vi "sicm_main.vi"(6 "sicm.blc.p.params":T8={"se.blc.p.postRetractDelay"=0, "se.blc.p.windowSize"=0, "se.blc.p.updateFactor"=-8, "blc.resetBackground"=FALSE, "se.blc.p.mindelta"=0.0}, 7 "sicm.display":T4, 8 "sicm.p.clocks":T10, 9 "sicm.p.params":T2={"sicm.p.setPoint"=0.9999847412109375, "sicm.p.setPointFrac"=1.0, "stepDown"=0.0, "retractHeight"=0.0, "adaptiveMin"=0.0} {"sicm.p.setPoint" format="%#_3g"}, 10 "sicm.p.modes":T9, 11 "sicm.i.current":T6) -> (0 "sicm.debug":T3, 1 "sicm.s.baseline":T1, 2 "sicm.triggerHeight":T7, 3 "heightOut":T5)   [LabVIEW 2016]
uses:
  <vilib>/rvi/FXPMathLib/FxpDiv/subVIs/nifxpmath_Div_SimConfig.ctl
  <vilib>/rvi/Emulation/niFpgaEmulationIsFPGAContextNoSignature.vi
  <vilib>/rvi/Emulation/niFpgaSctlEmulationGetInTimedLoop.vi
  <vilib>/rvi/errors/niFpgaSetErrorForExecOnDevCompSimple.vi
  <vilib>/rvi/eio/common/nirviEmuReportErrorAndStop.vi
  <vilib>/rvi/DataTransferAndStorage/Container/Common/niFpgaContainerGetUniqueNameForEmu.vi
  <vilib>/rvi/FIFO/Fifo_Resource/nirvififoEmulationSetSize.vi
  <vilib>/rvi/FIFO/Fifo_Resource/nirviFifoEmulationQueueMgr.vi
  <instcachedir>/0/nirviFifoEmulationQueueMgr_E5CAEC123FF24DC58D834DCA3CDAA9B5.lvgen/nirviFifoEmulationQueueMgr_E5CAEC123FF24DC58D834DCA3CDAA9B5_033.vi
  <vilib>/rvi/FIFO/Fifo_Resource/nirvififoEmulationDetermineInputValidOut.vi
  <vilib>/rvi/FIFO/Fifo_Resource/nirvififoEmulationCreateLock.vi
  <vilib>/rvi/Emulation/niFpgaProcessEmulError.vi
  <vilib>/rvi/FIFO/Fifo_Resource/nirvififoEmulationObtainLock.vi
  <vilib>/rvi/FIFO/Fifo_Resource/nirvififoEmulationReleaseLock.vi
  <vilib>/rvi/occurrence/nirviWaitOnOccurrenceBase.vi
  <vilib>/rvi/errors/nirviReportUnexpectedCaseInternalError.vi
  <vilib>/rvi/errors/nirviReportUnexpectedCaseInternalError (U32).vi
  <vilib>/rvi/FXPMathLib/FxpDiv/simVIs/DllFxpDivTemp_sub.vi
  <instrlib>/_niInstr/Basic Elements/v1/FPGA/Private/Count Down U8.vi
  <vilib>/rvi/FXPMathLib/FxpInterpret/XNode/nifxpmath_Interpret.xnode
  <vilib>/rvi/DataTransferAndStorage/Container/XNode/niFpgaContainer.xnode
  <vilib>/rvi/FIFO/Fifo_Resource/nirvififoEmulationWrite.vi
  <vilib>/rvi/FXPMathLib/FxpMul/XNode/nifxpmath_Multiplier.xnode
  <vilib>/rvi/FXPMathLib/FxpSub/XNode/nifxpmath_Sub.xnode
  <vilib>/rvi/FXPMathLib/FxpReciprocal/XNode/nifxpmath_Reciprocal.xnode
  <vilib>/rvi/FXPMathLib/FxpDiv/XNode/nifxpmath_Div.xnode
  <vilib>/rvi/DataTransferAndStorage/Handshake/Emulation/niFpgaHandshakeEmulation.vi
  <vilib>/rvi/FXPMathLib/FxpAdd/XNode/nifxpmath_Add.xnode
  <vilib>/rvi/FXPMathLib/sim/FxpSim.dll
  <instrlib>/_niInstr/Basic Elements/v1/FPGA/niInstr Basic Elements v1 FPGA.lvlib
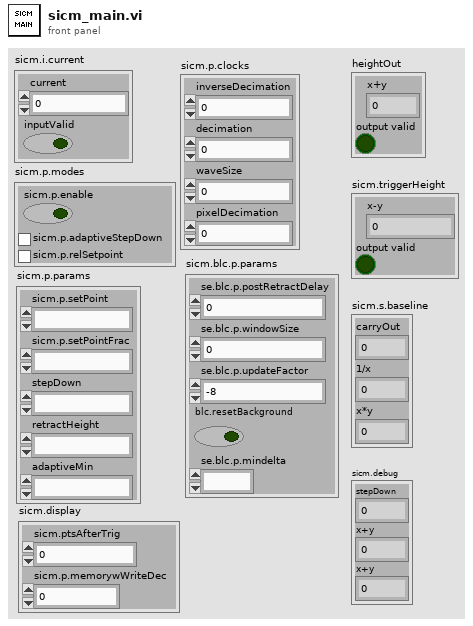
[diagram p1: front panel]
types:
  T1 = cluster{"carryOut":fxp<+/-,22,2>, "1/x":fxp<+/-,32,24>, "x*y":fxp<+,24,1>}
  T2 = cluster{"sicm.p.setPoint":fxp<+,20,0>, "sicm.p.setPointFrac":fxp<+/-,20,14>, "stepDown":fxp<+/-,28,4>, "retractHeight":fxp<+/-,28,4>, "adaptiveMin":fxp<+,10,0>}
  T3 = cluster{"stepDown":fxp<+/-,28,4>, "x+y":fxp<+/-,20,1>, "x+y":fxp<+/-,28,1>}
  T4 = cluster{"sicm.ptsAfterTrig":u16, "sicm.p.memorywWriteDec":u16}
  T5 = cluster{"x+y":fxp<+/-,28,2>, "output valid":bool}
  T6 = cluster{"current":fxp<+/-,24,16>, "inputValid":bool}
  T7 = cluster{"x-y":fxp<+/-,22,4>, "output valid":bool}
  T8 = cluster{"se.blc.p.postRetractDelay":u16, "se.blc.p.windowSize":u16, "se.blc.p.updateFactor":i16, "blc.resetBackground":bool, "se.blc.p.mindelta":fxp<+/-,12,-14>}
  T9 = cluster{"sicm.p.enable":bool, "sicm.p.adaptiveStepDown":bool, "sicm.p.relSetpoint":bool}
  T10 = cluster{"inverseDecimation":fxp<+,22,0>, "decimation":u16, "waveSize":u16, "pixelDecimation":u16}
  T11 = cluster{"address":u16, "interactionPair":cluster{"Current":i16, "Height":i16}}
  T12 = cluster{"upper limit":fxp<+/-,29,2>, "edge detected":bool}
  T13 = cluster{"current":fxp<+/-,24,16>, "y":fxp<+/-,29,16>}
  T14 = cluster{"carryOut":fxp<+/-,28,2>, "1/x":fxp<+/-,32,24>, "x*y":fxp<+,24,1>}
  T15 = cluster{"stepDown":fxp<+/-,28,4>, "upper limit":fxp<+/-,29,2>, "x+y":fxp<+/-,29,2>}
  T16 = cluster{"x+y":fxp<+/-,29,2>, "output valid":bool}
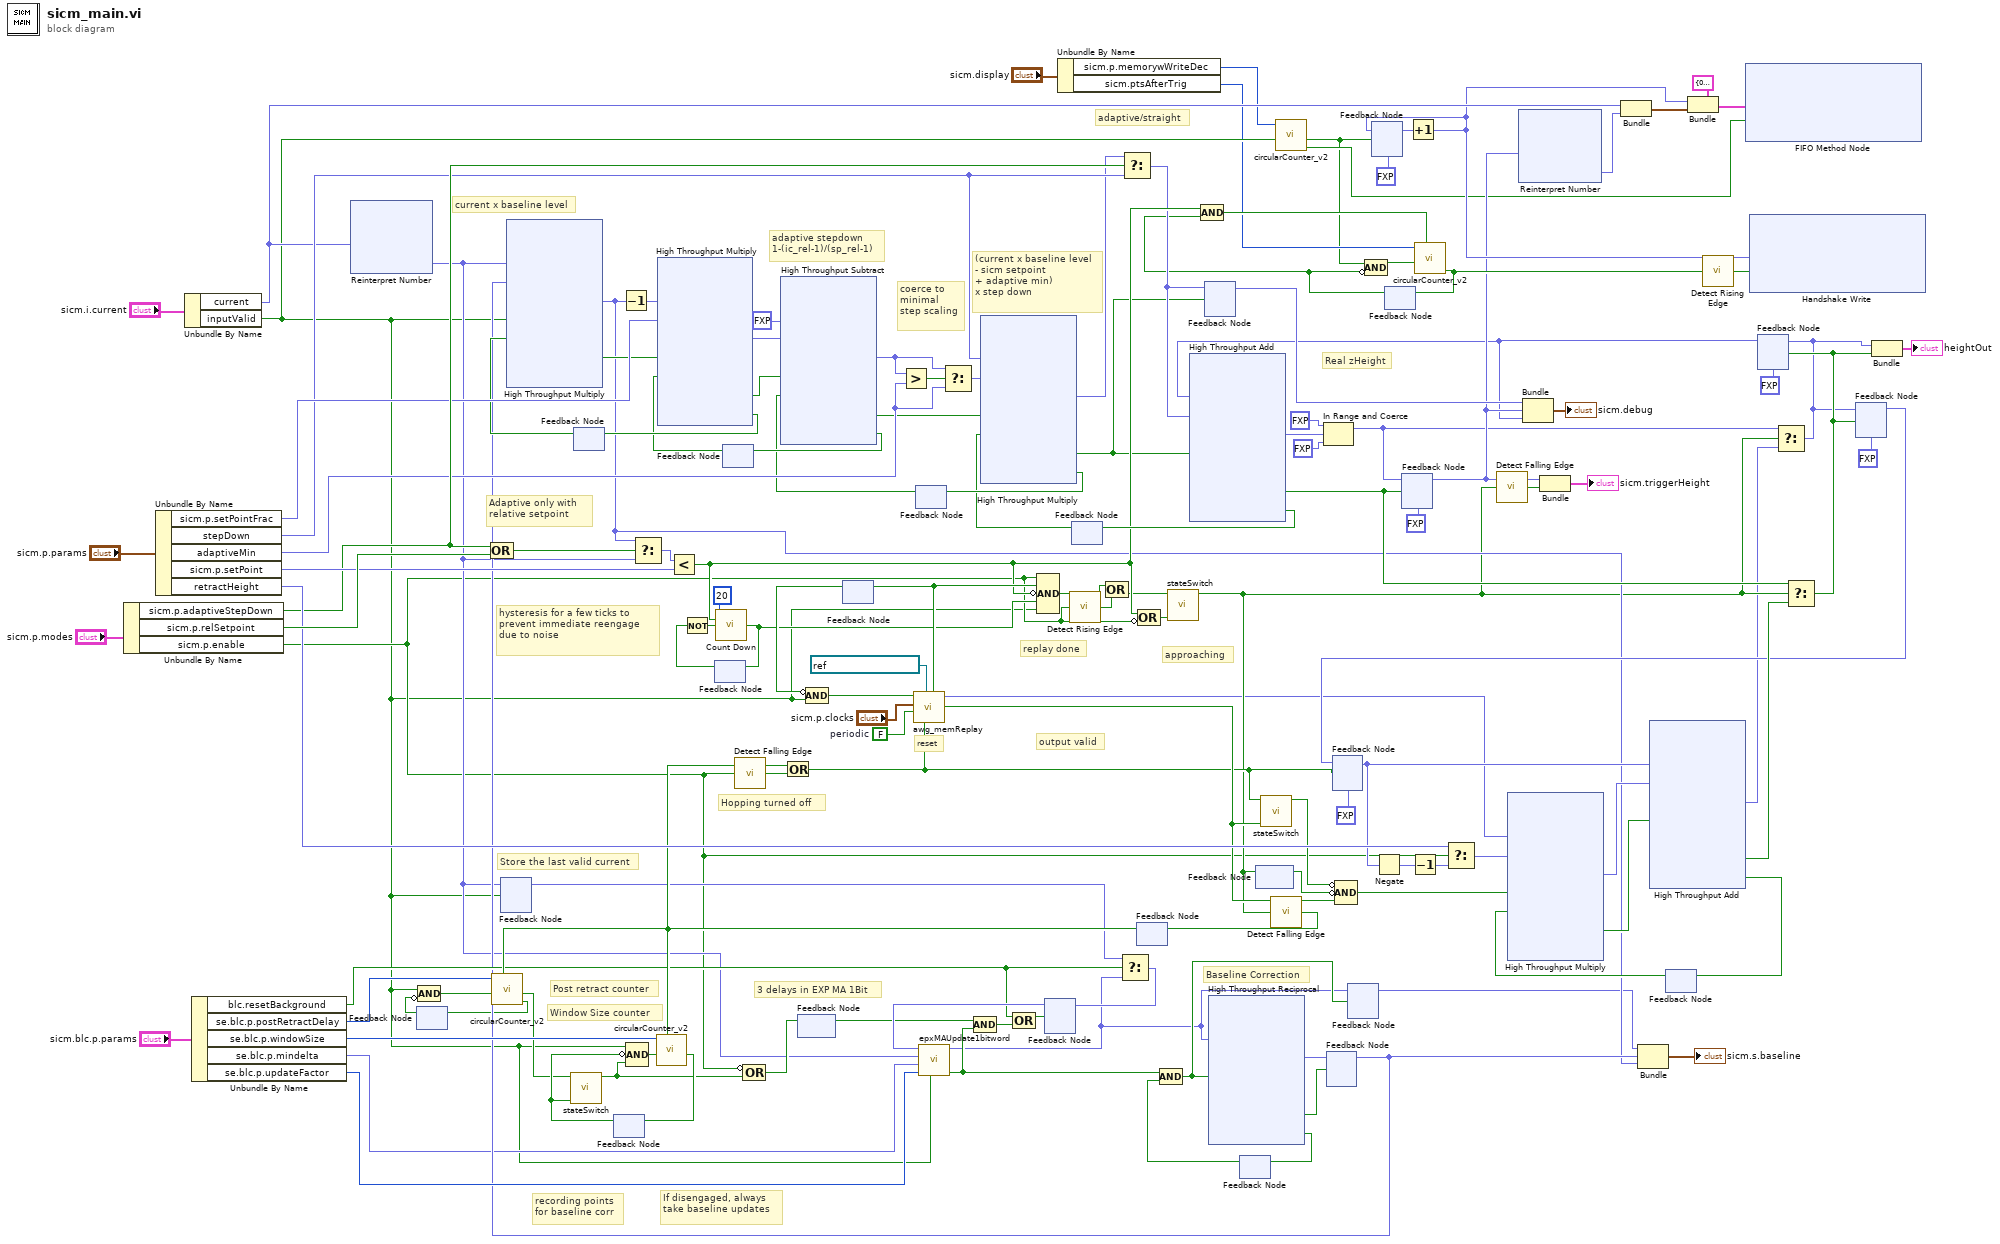
[diagram p0: block diagram]
diagram:
  w135 = FALSE  # periodic
  # "3 delays in EXP MA 1Bit"
  # "Window Size counter"
  # "Post retract counter"
  # "Hopping turned off"
  # "Store the last valid current"
  # "hysteresis for a few ticks to prevent immediate reengage due to noise"
  # "adaptive stepdown\n1-(ic_rel-1)/(sp_rel-1)"
  # "coerce to minimal step scaling"
  # "replay done"
  # "output valid"
  # "reset"
  # "(current x baseline level \n- sicm setpoint \n+ adaptive min)\nx step down"
  # "current x baseline level"
  # "If disengaged, always take baseline updates"
  # "Adaptive only with \nrelative setpoint"
  # "recording points\nfor baseline corr"
  # "Baseline Correction"
  # "adaptive/straight"
  # "approaching"
  # "Real zHeight"
  n1 = Unbundle By Name("sicm.p.modes") -> ("sicm.p.adaptiveStepDown"=w111:bool, "sicm.p.relSetpoint"=w120:bool, "sicm.p.enable"=w22:bool)
  n2 = Unbundle By Name("sicm.p.params") -> ("sicm.p.setPointFrac"=w104:fxp<+/-,20,14>, "stepDown"=w89:fxp<+/-,28,4>, "adaptiveMin"=w106:fxp<+,10,0>, "sicm.p.setPoint"=w115:fxp<+,20,0>, "retractHeight"=w114:fxp<+/-,28,4>)
  n3 = Unbundle By Name("sicm.i.current") -> ("current"=w64:fxp<+/-,24,16>, "inputValid"=w5:bool)
  n4 = Unbundle By Name("sicm.blc.p.params") -> ("blc.resetBackground"=w46:bool, "se.blc.p.postRetractDelay"=w118:u16, "se.blc.p.windowSize"=w117:u16, "se.blc.p.mindelta"=w19:fxp<+/-,12,-14>, "se.blc.p.updateFactor"=w116:i16)
  n5 = xnode "Reinterpret Number"("x"=w64) -> ("y"=w40:fxp<+/-,24,1>)
  n6 = feedback #1() -> (w75:bool)  [unwired: 1 in]
  n7 = Compound Arithmetic op=AND(w5, invert w75) -> (w76:bool)
  n8 = Compound Arithmetic op=OR(w111, w120) -> (w122:bool)
  n9 = feedback #2() -> (w49:fxp<+/-,24,1>)  [unwired: 1 in]
  n10 = feedback-in #2(w40, w5) -> ()
  n11 = feedback #3() -> (w98:bool)  [unwired: 1 in]
  n12 = feedback #4() -> (w52:bool)  [unwired: 1 in]
  n13 = feedback #5() -> (w70:bool)  [unwired: 1 in]
  n14 = Not(x=w70) -> (.not. x?=w69:bool)
  n15 = feedback #6() -> (w96:bool)  [unwired: 1 in]
  n16 = call <instrlib>:"Detect Falling Edge.vi"("signal"=w22) -> ("edge detected"=w130:bool)  [unwired: 14 in]
  n17 = feedback #7() -> (w12:bool)  [unwired: 1 in]
  n18 = feedback #8() -> (w80:bool)  [unwired: 1 in]
  n19 = Compound Arithmetic op=AND(invert w80, w5) -> (w110:bool)
  n20 = feedback #9() -> (w94:bool)  [unwired: 1 in]
  n21 = feedback #10() -> (w127:fxp<+/-,28,2>)  [unwired: 1 in]
  n22 = call "epxMAUpdate1bitword.vi"("input valid"=w5, "expFactor"=w116, "min delta"=w19, "update"=w40, "carryIn"=w127) -> ("output valid"=w38:bool, "carryOut"=w15:fxp<+/-,28,2>)  [unwired: 5 in]
  n23 = Compound Arithmetic op=AND(w12, w38) -> (w47:bool)
  n24 = Compound Arithmetic op=OR(w46, w47) -> (w48:bool)
  n25 = Unbundle By Name("sicm.display") -> ("sicm.p.memorywWriteDec"=w2:u16, "sicm.ptsAfterTrig"=w3:u16)
  n26 = call <instrlib>:"Detect Rising Edge.vi"("signal"=w22) -> ("edge detected"=w21:bool)  [unwired: 14 in]
  n27 = feedback #11() -> (w85:bool)  [unwired: 1 in]
  n28 = Select(t=w49, s=w46, f=w15) -> (s? t:f=w50:fxp<+/-,28,2>)
  n29 = feedback-in #10(w50, w48) -> ()
  n30 = feedback #12() -> (w84:bool)  [unwired: 1 in]
  n31 = call "circularCounter_v2.vi"("reset"=w84, "doStep"=w76, "maxCount"=w118) -> ("maxReached"=w37:bool, "maxPulse"=w36:bool)  [unwired: 5 in, 2 out]
  n32 = feedback-in #1(w37) -> ()
  n33 = call "stateSwitch.vi"("disable"=w52, "enable"=w36) -> ("state"=w13:bool)  [unwired: 9 in]
  n34 = Compound Arithmetic op=AND(w5, invert w52, w13) -> (w74:bool)
  n35 = call "circularCounter_v2.vi"("reset"=w84, "doStep"=w74, "maxCount"=w117) -> ("maxPulse"=w128:bool)  [unwired: 5 in, 3 out]
  n36 = feedback-in #4(w128) -> ()
  n37 = Compound Arithmetic op=OR(invert w22, w13) -> (w139:bool)
  n38 = Or(x=w84, y=w130) -> (x .or. y?=w77:bool)
  n39 = feedback-in #7(w139) -> ()
  n40 = call "awg_memReplay.vi"("reset"=w77, "memSelector"=refnum<k21> "sicm.upMotion", "periodic"=w135, "clocks"="sicm.p.clocks", "output"=w110) -> ("outputValid"=w78:bool, "interpOutput"=w32:fxp<+/-,19,2>, "replayDone"=w90:bool)  [unwired: 2 in, 2 out]
  n41 = feedback-in #8(w90) -> ()
  n42 = feedback #13() -> (w28:fxp<+/-,28,4>)  [unwired: 1 in]
  n43 = feedback #14() -> (w51:bool)  [unwired: 1 in]
  n44 = Compound Arithmetic op=AND(w38, w51) -> (w16:bool)
  n45 = xnode "High Throughput Reciprocal"("x"=w15, "input valid"=w16) -> ("1/x"=w124:fxp<+/-,32,24>, "output valid"=w125:bool, "ready for input"=w126:bool)  [unwired: 1 in]
  n46 = feedback-in #14(w126) -> ()
  n47 = feedback #15() -> (w82:bool)  [unwired: 1 in]
  n48 = call "stateSwitch.vi"("disable"=w78, "enable"=w77) -> ("state"=w79:bool)  [unwired: 9 in]
  n49 = call "circularCounter_v2.vi"("doStep"=w5, "maxCount"=w2) -> ("maxReached"=w4:bool, "maxPulse"=w1:bool)  [unwired: 6 in, 2 out]
  n50 = feedback #16() -> (w42:fxp<+/-,32,24>)  [unwired: 1 in]
  n51 = xnode ("High Throughput Multiply")("x"=w40, "y"=w42, "input valid"=w5, "ready for output (T)"=w98) -> ("x*y"=w41:fxp<+,24,1>, "output valid"=w103:bool)  [unwired: 1 out]
  n52 = Decrement(x=w41) -> (x-1=w105:fxp<+/-,24,1>)
  n53 = Select(t=w41, s=w122, f=w40) -> (s? t:f=w123:fxp<+/-,25,2>)
  n54 = xnode ("High Throughput Multiply")("x"=w105, "y"=w104, "input valid"=w103, "ready for output (T)"=w96) -> ("x*y"=w101:fxp<+/-,24,4>, "output valid"=w100:bool, "ready for input"=w99:bool)
  n55 = feedback-in #3(w99) -> ()
  n56 = Less?(x=w123, y=w115) -> (x < y?=w61:bool)
  n57 = call-poly <instrlib>:"Count Down.vi"("count in"=u8 20, "load"=w61, "decrement"=w69) -> ("terminal count"=w67:bool)  [unwired: 11 in, 1 out]
  n58 = feedback-in #5(w67) -> ()
  n59 = xnode "High Throughput Subtract"("x"=fxp<+,1,1> 1.0, "y"=w101, "input valid"=w100, "ready for output (T)"=w94) -> ("x-y"=w92:fxp<+/-,22,4>, "output valid"=w95:bool, "ready for input"=w97:bool)
  n60 = feedback-in #6(w97) -> ()
  n61 = Greater?(x=w92, y=w106) -> (0:w107:bool)
  n62 = Select(t=w92, s=w107, f=w106) -> (s? t:f=w87:fxp<+/-,22,4>)
  n63 = xnode ("High Throughput Multiply")("x"=w89, "y"=w87, "input valid"=w95, "ready for output (T)"=w85) -> ("x*y"=w88:fxp<+/-,28,4>, "output valid"=w29:bool, "ready for input"=w138:bool)
  n64 = feedback-in #9(w138) -> ()
  n65 = Compound Arithmetic op=AND(w22, w90, invert w61, w67, w5) -> (w20:bool)
  n66 = Compound Arithmetic op=OR(w20, w21) -> (w23:bool)
  n67 = Select(t=w88, s=w111, f=w89) -> (s? t:f=w30:fxp<+/-,28,4>)
  n68 = Compound Arithmetic op=OR(w61, invert w22) -> (w34:bool)
  n69 = call "stateSwitch.vi"("disable"=w34, "enable"=w23) -> ("state"=w35:bool)  [unwired: 9 in]
  n70 = feedback-in #13(w30, w29) -> ()
  n71 = feedback-in #15(w35) -> ()
  n72 = call <instrlib>:"Detect Falling Edge.vi"("signal"=w35) -> ("edge detected"=w129:bool)  [unwired: 14 in]
  n73 = feedback-in #12(w129) -> ()
  n74 = feedback-in #16(w124, w125) -> ()
  n75 = feedback #17(fxp<+/-,28,1> -1.0 ("x-y")) -> (w81:fxp<+/-,29,2>)
  n76 = Compound Arithmetic op=AND(invert w79, invert w82, w78) -> (w83:bool)
  n77 = feedback #18() -> (w14:fxp<+/-,28,2>)  [unwired: 1 in]
  n78 = feedback-in #18(w15, w16) -> ()
  n79 = feedback #19(fxp<+,14,14> 0.0) -> (w62:fxp<+,14,14>)
  n80 = Negate(x=w81) -> (-x=w109:fxp<+/-,30,3>)
  n81 = feedback #20() -> (w17:bool)  [unwired: 1 in]
  n82 = Compound Arithmetic op=AND(w61, w17) -> (w18:bool)
  n83 = Compound Arithmetic op=AND(w1, invert w17) -> (w53:bool)
  n84 = feedback #21(fxp<+/-,28,1> -1.0 ("x+y")) -> (w27:fxp<+/-,29,2>)
  n85 = Increment(x=w62) -> (x+1=w58:fxp<+,14,14>)
  n86 = feedback-in #19(w58, w1) -> ()
  n87 = Decrement(x=w109) -> (x-1=w91:fxp<+/-,30,3>)
  n88 = call "circularCounter_v2.vi"("reset"=w18, "doStep"=w53, "maxCount"=w3) -> ("maxReached"=w55:bool)  [unwired: 5 in, 3 out]
  n89 = feedback-in #20(w55) -> ()
  n90 = Select(t=w114, s=w22, f=w91) -> (s? t:f=w33:fxp<+/-,31,4>)
  n91 = call <instrlib>:"Detect Falling Edge.vi"("signal"=w35) -> ("edge detected"=w71:bool)  [unwired: 14 in]
  n92 = xnode "Reinterpret Number"("x"=w27) -> ("y"=w57:fxp<+/-,29,16>)
  n93 = Bundle("upper limit"=w27, "edge detected"=w71) -> (→"sicm.triggerHeight":T12)  [unwired: 1 in]
  n94 = Bundle("current"=w64, "y"=w57) -> (w65:T13)  [unwired: 1 in]
  n95 = Bundle("carryOut"=w14, "1/x"=w42, "x*y"=w41) -> (→"sicm.s.baseline":T14)  [unwired: 1 in]
  n96 = feedback #22() -> (w131:bool)  [unwired: 1 in]
  n97 = xnode ("High Throughput Multiply")("x"=w32, "y"=w33, "input valid"=w83, "ready for output (T)"=w131) -> ("x*y"=w59:fxp<+/-,21,3>, "output valid"=w134:bool)  [unwired: 1 out]
  n98 = xnode ("High Throughput Add")("x"=w81, "y"=w59, "input valid"=w134) -> ("x+y"=w31:fxp<+/-,28,1>, "output valid"=w133:bool, "ready for input"=w132:bool)  [unwired: 1 in]
  n99 = feedback-in #22(w132) -> ()
  n100 = Bundle(cluster=T11 {"address"=0, "interactionPair"={"Current"=0, "Height"=0}} ("Element"), "address"=w58, "interactionPair"=w65) -> (w56:T11)
  n101 = call <instrlib>:"Detect Rising Edge.vi"("signal"=w55) -> ("edge detected"=w54:bool)  [unwired: 14 in]
  n102 = xnode ("FIFO Method Node")("Element"=w56, "Input Valid"=w4) -> ()  [unwired: 1 in, 2 out]
  n103 = xnode ("Handshake Write")("Data"=w58, "Input Valid"=w54) -> ()  [unwired: 1 in, 2 out]
  n104 = feedback #23(fxp<+/-,28,1> -1.0 ("x+y")) -> (w26:fxp<+/-,29,2>)
  n105 = xnode ("High Throughput Add")("x"=w26, "y"=w30, "input valid"=w29) -> ("x+y"=w93:fxp<+/-,28,2>, "output valid"=w73:bool, "ready for input"=w86:bool)  [unwired: 1 in]
  n106 = feedback-in #11(w86) -> ()
  n107 = In Range and Coerce(upper limit=fxp<+/-,28,2> 1.0, x=w93, lower limit=fxp<+/-,28,2> -1.0 ("x")) -> (coerced(x)=w8:fxp<+/-,28,2>)  [unwired: 1 out]
  n108 = feedback-in #21(w8, w73) -> ()
  n109 = Bundle("stepDown"=w28, "upper limit"=w27, "x+y"=w26) -> (→"sicm.debug":T15)  [unwired: 1 in]
  n110 = Select(t=w8, s=w35, f=w31) -> (s? t:f=w39:fxp<+/-,29,2>)
  n111 = Select(t=w73, s=w35, f=w133) -> (s? t:f=w45:bool)
  n112 = feedback-in #23(w39, w45) -> ()
  n113 = feedback #24(fxp<+/-,28,1> -1.0 ("x+y")) -> (w44:fxp<+/-,29,2>)
  n114 = feedback-in #17(w44, w77) -> ()
  n115 = feedback-in #24(w39, w45) -> ()
  n116 = Bundle("x+y"=w39, "output valid"=w45) -> (→"heightOut":T16)  [unwired: 1 in]
